vi "SimulateTemperature.vi"(1 "TimeSeconds":dbl, 2 "NoiseAmp":dbl=2.0, 3 "BaseTemp":dbl=25.0) -> (0 "Temp Out":dbl)   [LabVIEW 2025]
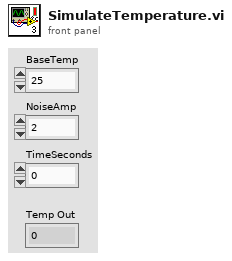
[diagram p1: front panel]
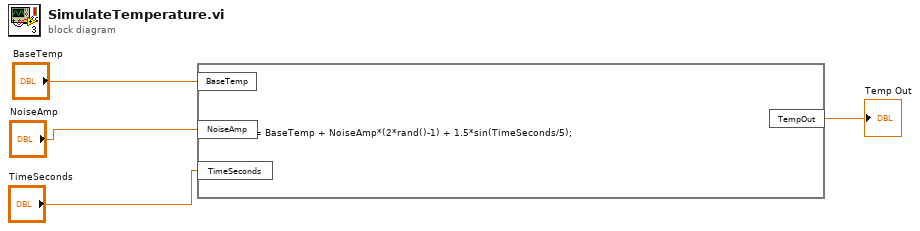
[diagram p0: block diagram]
diagram:
  n1 = formula code="TempOut = BaseTemp + NoiseAmp*(2*rand()-1) + 1.5*sin(TimeSeconds/5);"("BaseTemp"="BaseTemp", "NoiseAmp"="NoiseAmp", "TimeSeconds"="TimeSeconds") -> ("TempOut"=→"Temp Out":dbl)
